vi "M07 Energy Cells.vi"(11 "NXT/EV3":T1) -> ()   [LabVIEW 2016]
uses:
  <vilib>/NXT/Subs/LVHSConnector.ctl
  <vilib>/NXT/LegoClasses/BrickReference/BrickReference.lvclass
  <vilib>/NXT/Block Support/NXT_InputPort.ctl
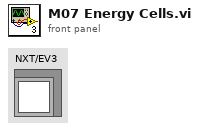
[diagram p1: front panel]
types:
  T1 = typedef "LVHSConnector.ctl" = refnum<class "BrickReference.lvclass">
  T2 = typedef "NXT_InputPort.ctl" = u32
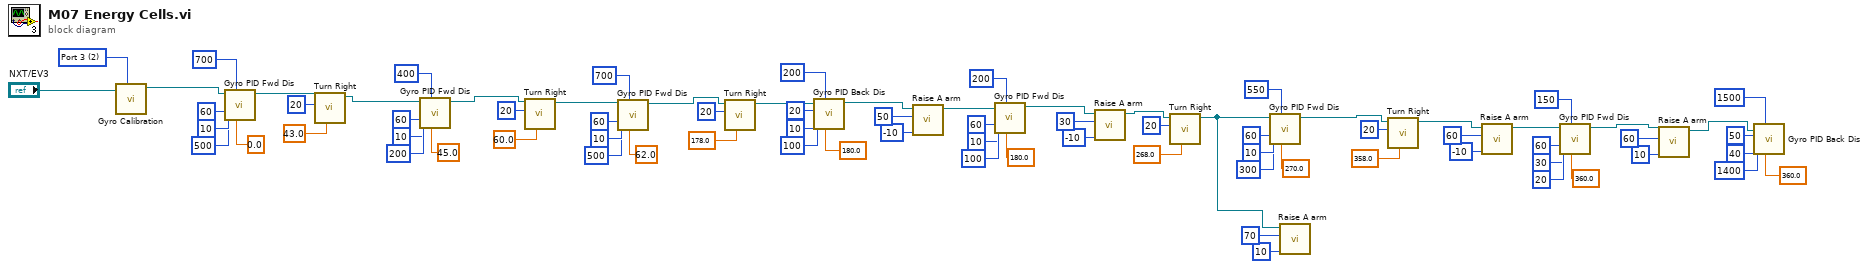
[diagram p0: block diagram]
diagram:
  w73 = T2 2 items=["Port 1", "Port 2", "Port 3", "Port 4"] ("Port (Port 1)")
  n1 = call "Gyro Calibration.vi"("Port (Port 1)"=w73, "NXT/EV3"="NXT/EV3") -> ("NXT/EV3"=w74:T1)  [unwired: 5 in, 2 out]
  n2 = call "Gyro PID Fwd Dis.vi"("Target angle"=sgl 0.0, "Threshold to stop"=700, "Threshold to slow"=500, "Min. speed"=10, "Max. speed"=60, "EV3 in"=w74) -> ("EV3 out"=w71:T1)  [unwired: 5 in]
  n3 = call "Turn Right.vi"("Turning angle"=sgl 43.0, "Motor B (right)"=i8 20, "EV3 in"=w71) -> ("EV3 out"=w63:T1)  [unwired: 8 in]
  n4 = call "Gyro PID Fwd Dis.vi"("Target angle"=sgl 45.0, "Threshold to stop"=400, "Threshold to slow"=200, "Min. speed"=10, "Max. speed"=60, "EV3 in"=w63) -> ("EV3 out"=w60:T1)  [unwired: 5 in]
  n5 = call "Turn Right.vi"("Turning angle"=sgl 60.0, "Motor B (right)"=i8 20, "EV3 in"=w60) -> ("EV3 out"=w54:T1)  [unwired: 8 in]
  n6 = call "Gyro PID Fwd Dis.vi"("Target angle"=sgl 62.0, "Threshold to stop"=700, "Threshold to slow"=500, "Min. speed"=10, "Max. speed"=60, "EV3 in"=w54) -> ("EV3 out"=w51:T1)  [unwired: 5 in]
  n7 = call "Turn Right.vi"("Turning angle"=sgl 178.0, "Motor B (right)"=i8 20, "EV3 in"=w51) -> ("EV3 out"=w50:T1)  [unwired: 8 in]
  n8 = call "Gyro PID Back Dis.vi"("Target angle"=sgl 180.0, "Threshold to stop"=200, "Threshold to slow"=100, "Min. speed"=10, "Max. speed"=20, "EV3 in"=w50) -> ("EV3 out"=w42:T1)  [unwired: 5 in]
  n9 = call "Raise A arm.vi"("Power"=i8 -10, "Rotation"=50, "EV3 in"=w42) -> ("EV3 out"=w36:T1)  [unwired: 8 in]
  n10 = call "Gyro PID Fwd Dis.vi"("Target angle"=sgl 180.0, "Threshold to stop"=200, "Threshold to slow"=100, "Min. speed"=10, "Max. speed"=60, "EV3 in"=w36) -> ("EV3 out"=w33:T1)  [unwired: 5 in]
  n11 = call "Raise A arm.vi"("Power"=i8 -10, "Rotation"=30, "EV3 in"=w33) -> ("EV3 out"=w30:T1)  [unwired: 8 in]
  n12 = call "Turn Right.vi"("Turning angle"=sgl 268.0, "Motor B (right)"=i8 20, "EV3 in"=w30) -> ("EV3 out"=w22:T1)  [unwired: 8 in]
  n13 = call "Gyro PID Fwd Dis.vi"("Target angle"=sgl 270.0, "Threshold to stop"=550, "Threshold to slow"=300, "Min. speed"=10, "Max. speed"=60, "EV3 in"=w22) -> ("EV3 out"=w19:T1)  [unwired: 5 in]
  n14 = call "Raise A arm.vi"("Power"=i8 10, "Rotation"=70, "EV3 in"=w22) -> ()  [unwired: 8 in, 1 out]
  n15 = call "Turn Right.vi"("Turning angle"=sgl 358.0, "Motor B (right)"=i8 20, "EV3 in"=w19) -> ("EV3 out"=w16:T1)  [unwired: 8 in]
  n16 = call "Raise A arm.vi"("Power"=i8 -10, "Rotation"=60, "EV3 in"=w16) -> ("EV3 out"=w10:T1)  [unwired: 8 in]
  n17 = call "Gyro PID Fwd Dis.vi"("Target angle"=sgl 360.0, "Threshold to stop"=150, "Threshold to slow"=20, "Min. speed"=30, "Max. speed"=60, "EV3 in"=w10) -> ("EV3 out"=w7:T1)  [unwired: 5 in]
  n18 = call "Raise A arm.vi"("Power"=i8 10, "Rotation"=60, "EV3 in"=w7) -> ("EV3 out"=w1:T1)  [unwired: 8 in]
  n19 = call "Gyro PID Back Dis.vi"("Target angle"=sgl 360.0, "Threshold to stop"=1500, "Threshold to slow"=1400, "Min. speed"=40, "Max. speed"=50, "EV3 in"=w1) -> ()  [unwired: 5 in, 1 out]
